vi "AlliGator Get Hot Pixel Removal String.vi"(8 "Error In":errorcluster, 11 "Hot Pixel Removal":T1 {"Percentile" min=0 max=100}) -> (0 "Error Out":errorcluster, 3 "String":string)   [LabVIEW 2021, in "AlliGator Source Image.lvlib"]
doc: "Builds string describing hot pixel removal options."
uses:
  AlliGator Source Image.lvlib
  SwissSPAD/SwissSPAD Live_Image Display Options.ctl
  SwissSPAD/SwissSPAD Live.lvlib
panel:
  # "see the AlliGator License on the block diagram (Ctrl+E or Window:Show Block Diagram)"
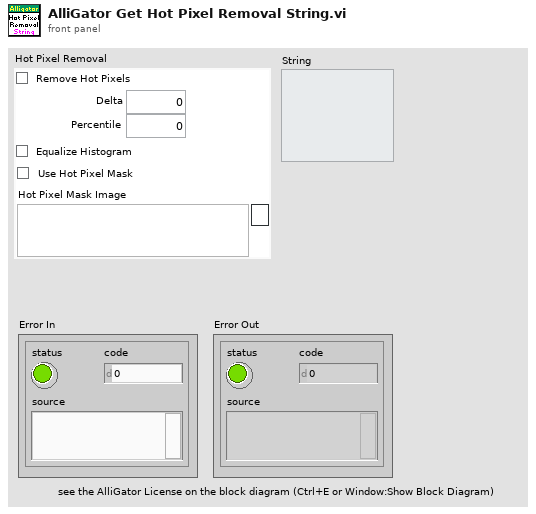
[diagram p1: front panel]
types:
  T1 = typedef "SwissSPAD Live.lvlib/SwissSPAD Live_Image Display Options.ctl" = cluster{"Remove Screamers":bool, "Delta":sgl, "Equalize Histogram":bool, "Percentile":sgl, "Hot Pixel Mask Image":path, "Use Hot Pixel Mask":bool}
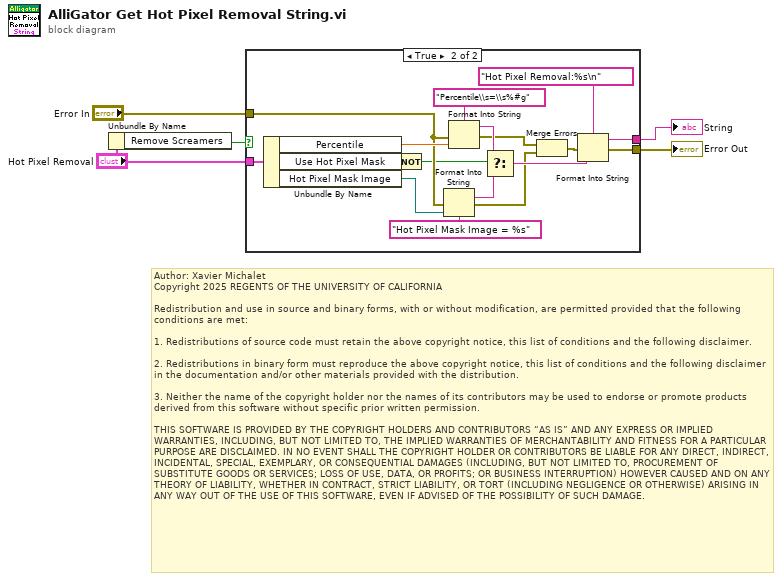
[diagram p0: block diagram]
diagram:
  # "Author: Xavier Michalet\nCopyright 2025 REGENTS OF THE UNIVERSITY OF CALIFORNIA\n\nRedistribution and use in source and binary forms, with or without modification, are permitted provided that the following conditions are met:\n\n1. Redistributions of source code must retain the above copyright notice, this list of conditions and the following disclaimer.\n\n2. Redistributions in binary form must reproduce the above copyright notice, this list of conditions and the following disclaimer in the documentation and/or other materials provided with the distribution.\n\n3. Neither the name of the copyright holder nor the names of its contributors may be used to endorse or promote products derived from this software without specific prior written permission.\n\nTHIS SOFTWARE IS PROVIDED BY THE COPYRIGHT HOLDERS AND CONTRIBUTORS “AS IS” AND ANY EXPRESS OR IMPLIED WARRANTIES, INCLUDING, BUT NOT LIMITED TO, THE IMPLIED WARRANTIES OF MERCHANTABILITY AND FITNESS FOR A PARTICULAR PURPOSE ARE DISCLAIMED. IN NO EVENT SHALL THE COPYRIGHT HOLDER OR CONTRIBUTORS BE LIABLE FOR ANY DIRECT, INDIRECT, INCIDENTAL, SPECIAL, EXEMPLARY, OR CONSEQUENTIAL DAMAGES (INCLUDING, BUT NOT LIMITED TO, PROCUREMENT OF SUBSTITUTE GOODS OR SERVICES; LOSS OF USE, DATA, OR PROFITS; OR BUSINESS INTERRUPTION) HOWEVER CAUSED AND ON ANY THEORY OF LIABILITY, WHETHER IN CONTRACT, STRICT LIABILITY, OR TORT (INCLUDING NEGLIGENCE OR OTHERWISE) ARISING IN ANY WAY OUT OF THE USE OF THIS SOFTWARE, EVEN IF ADVISED OF THE POSSIBILITY OF SUCH DAMAGE."
  n1 = Unbundle By Name("Hot Pixel Removal") -> ("Remove Screamers"=w3:bool)
  n2 = case shown="True" w3 {
    tunnel: [_ w23] -> w5
    tunnel: "Hot Pixel Removal" -> [_ w20]
    tunnel: "Error In" -> [w6 w15]
    tunnel: [w6 w22] -> w1
    frame False {
    }
    frame True {
      n3 = Unbundle By Name(w20) -> ("Percentile"=w19:sgl, "Use Hot Pixel Mask"=w14:bool, "Hot Pixel Mask Image"=w16:path)
      n4 = Not(x=w14) -> (.not. x?=w13:bool)
      n5 = Format Into String(format string="Hot Pixel Mask Image = %s", error in=w15, w16) -> (resulting string=w11:string, error out=w7:errorcluster)  [unwired: 1 in]
      n6 = Format Into String(format string="Percentile\\s=\\s%#g", error in=w15, w19) -> (resulting string=w12:string, error out=w9:errorcluster)  [unwired: 1 in]
      n7 = Select(t=w12, s=w13, f=w11) -> (s? t:f=w10:string)
      n8 = Merge Errors(w9, w7) -> (w8:errorcluster)
      n9 = Format Into String(format string="Hot Pixel Removal:%s\n", error in=w8, w10) -> (resulting string=w23:string, error out=w22:errorcluster)  [unwired: 1 in]
    }
  }
  "String" <- w5
  "Error Out" <- w1
